vi "Database Command Create Parameters.vi"(8 "error in (no error)":errorcluster caption="错误输入（无错误）", 9 "parameters":T1[](array[typedef]), 11 "Database Command 输入":refnum<class "Database Command.lvclass"> caption="DNL_LabVIEW Object in") -> (0 "error out":errorcluster caption="错误输出", 3 "Database Command 输出":refnum<class "Database Command.lvclass"> caption="DNL_LabVIEW Object out")   [LabVIEW 2011, in "Database Command.lvclass"]
uses:
  Database Command.lvclass
  <vilib>/addons/database/Auxilliary.llb/DB Tools Parameter Info.ctl
  <vilib>/addons/database/Auxilliary.llb/DB Tools DataTypes.ctl
  <vilib>/addons/database/Auxilliary.llb/DB Tools Parameter Dir.ctl
  Database Command.lvclass/Database Command.ctl
  <vilib>/addons/database/NI_Database_API.lvlib
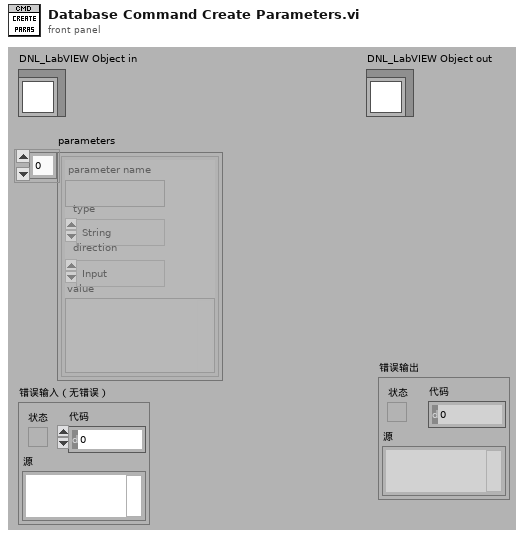
[diagram p1: front panel]
types:
  T1 = typedef "NI_Database_API.lvlib/DB Tools Parameter Info.ctl" = cluster{"parameter name":string, "type":T2, "direction":T3, "value":variant}
  T2 = typedef "NI_Database_API.lvlib/DB Tools DataTypes.ctl" = enum16{"String", "Long (I32)", "Single (SGL)", "Double (DBL)", "Date/Time", "Binary"}
  T3 = typedef "NI_Database_API.lvlib/DB Tools Parameter Dir.ctl" = enum32{"Input", "Output", "Input/Output", "Return Value"}
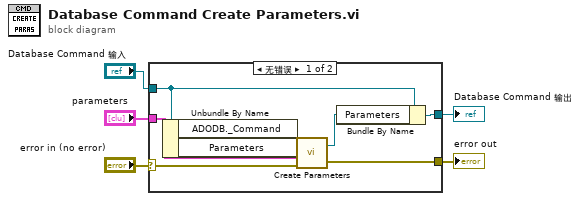
[diagram p0: block diagram]
diagram:
  n1 = case shown="无错误" "error in (no error)" {
    selector: "error in (no error)" -> [w12 _]
    tunnel: [w8 w14] -> w3
    tunnel: "Database Command 输入" -> [w7 w14]
    tunnel: "parameters" -> [w13 _]
    tunnel: [w11 _] -> w1
    frame No Error {
      n2 = Unbundle By Name(w7) -> ("ADODB._Command"=w10:refnum<k7>, "Parameters"=w9:refnum<k7>)
      n3 = call "Create Parameters.vi"("error IO"=w12, "parameters"=w13, "Parameters in"=w9, "ADODB._Command"=w10) -> ("error out"=w11:errorcluster, "Parameters out"=w6:refnum<k7>)
      n4 = Bundle By Name(cluster=w7, "Parameters"=w6) -> (w8:refnum<class "Database Command.lvclass">)
    }
    frame Error {
    }
  }
  "error out" <- w1
  "Database Command 输出" <- w3
